vi "Ctor.vi"(8 "error in (no error)":errorcluster, 11 "Square Field Panel in":refnum<class "Square Field Panel.lvclass">) -> (0 "error out":errorcluster, 3 "Square Field Panel out":refnum<class "Square Field Panel.lvclass">)   [LabVIEW 2020, in "SB App.lvlib" / "Square Field Panel.lvclass"]
uses:
  Square Field Panel.lvclass
  Square Map Update Data.ctl
  Square Field Panel.lvclass/Square Field Panel.ctl
  <vilib>/IlluminatedG/IG OOPanel/OOPanel/Panel/Panel.lvclass
  SB App.lvlib
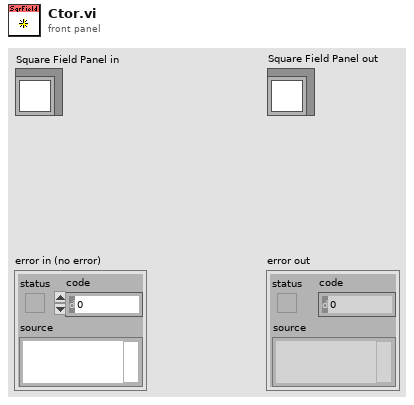
[diagram p1: front panel]
types:
  T1 = typedef "SB App.lvlib/Square Map Update Data.ctl" = cluster{"Square Color Map":u32[][]}
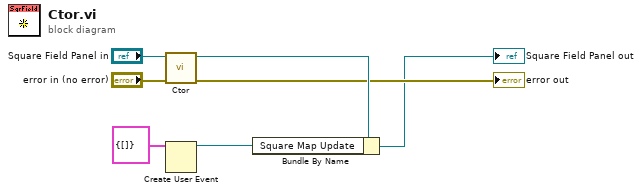
[diagram p0: block diagram]
diagram:
  n1 = call-parent "Ctor.vi"("error in (no error)"="error in (no error)", "Panel in"="Square Field Panel in") -> ("error out"=→"error out":errorcluster, "Panel out"=w5:refnum<class "Square Field Panel.lvclass">)  [unwired: 8 in]
  n2 = Create User Event(user event datatype=T1 {"Square Color Map"=[]} ("Square Map Update Data")) -> (user event=w1:refnum<user-event>)  [unwired: 1 in, 1 out]
  n3 = Bundle By Name(cluster=w5, "Square Map Update"=w1) -> (→"Square Field Panel out":refnum<class "Square Field Panel.lvclass">)
